vi "scandata.vi"() -> ()   [LabVIEW 2020]
uses:
  <userlib>/Nanonis Prog Interface V5/Nanonis Prog Interface.lvlib
panel:
  in  "function name":string
  in  "module path":path
  in  "Y (m)":sgl min=-0.001 max=0.001 format="%.3p"
  in  "X (m)":sgl min=-0.001 max=0.001 format="%.3p"
  in  "Center coordinates (m)":cluster{"Xc":sgl, "Yc":sgl}={"Xc"=nan, "Yc"=nan} caption="Center coordinates (m) (NaN=no change)" {"Yc" format="%.2p"; "Xc" format="%.2p"}
  in  "Pixels":i32 caption="Pixels/line (0=no change)"
  out "Lines":i32
  out "Pixels/line":i32
  out "Channels indexes (0-23)":i32[](array[numeric])
  in  "Auto save":bool
  in  "Serie name":string="ScanMultiBias_"
  in  "Bias increment":sgl=0.1
  in  "Number of scans":u8=5
  out "Bias voltage":sgl caption="Current bias voltage"
  out "Scan":u8 caption="Current scan"
  out "Saved file path":path
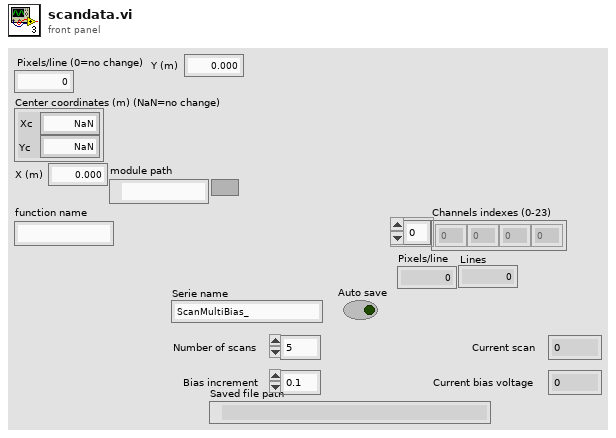
[diagram p1: front panel]
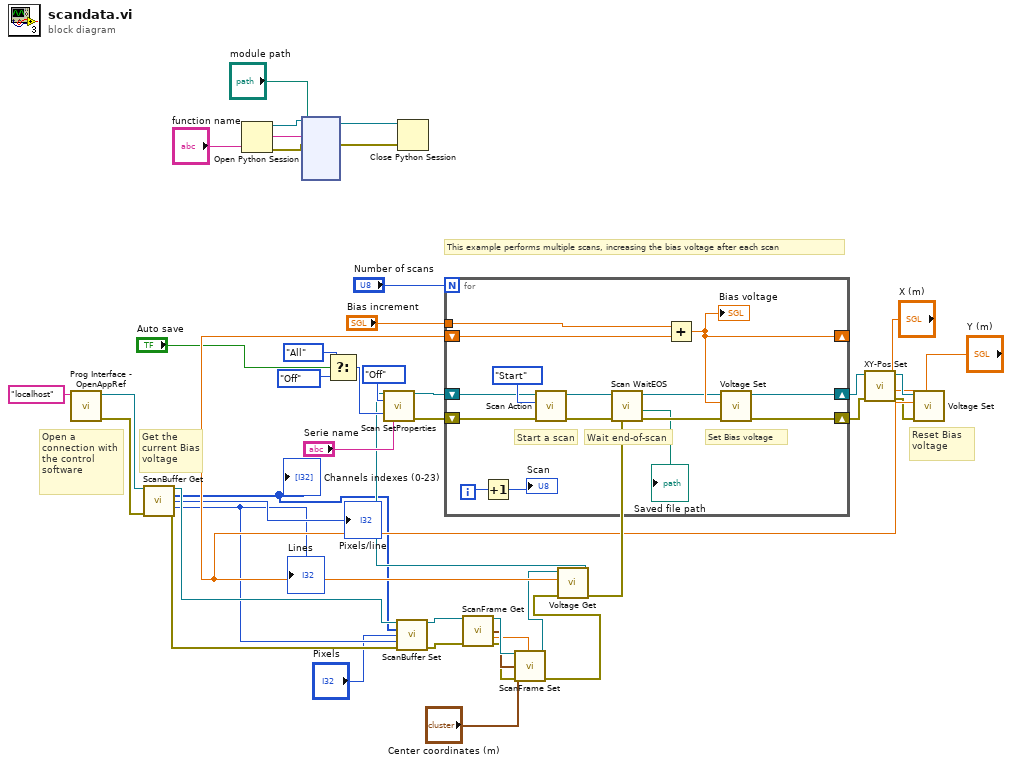
[diagram p0: block diagram]
diagram:
  # "Reset Bias voltage"
  # "Open a connection with the control\nsoftware"
  # "This example performs multiple scans, increasing the bias voltage after each scan"
  # "Get the current Bias voltage"
  n1 = call <userlib>:"Prog Interface - OpenAppRef.vi"("Machine name (local machine IP)"="localhost" ("Machine name (localhost)")) -> ("Error out"=w29:errorcluster, "Application reference"=w28:refnum<vi>)  [unwired: 5 in]
  n2 = call <userlib>:"ScanBuffer Get.vi"("Application ref in"=w28, "error in (no error)"=w29) -> ("Application ref out"=w27:refnum<vi>, "Channels indexes (0-23)"=w25:i32[], "Pixels/line"=→"Pixels/line":i32, "Lines"=w23:i32, "error out"=w26:errorcluster)  [unwired: 9 in]
  "Channels indexes (0-23)" <- w25
  "Lines" <- w23
  n3 = Open Python Session() -> (session out=w6:refnum<k35>, error out=w2:errorcluster)  [unwired: 3 in]
  n4 = node(w6, "module path", "function name", w2) -> (w4:refnum<k35>, w3:errorcluster)  [unwired: 8 in, 2 out]
  n5 = Select(t=enum16{"No change", "All", "Next", "Off"}."All" ("Auto save"), s="Auto save", f=enum16{"No change", "All", "Next", "Off"}."Off" ("Auto save")) -> (s? t:f=w32:enum16{"No change", "All", "Next", "Off"})
  n6 = call <userlib>:"ScanBuffer Set.vi"("Application ref in"=w27, "Channels indexes (0-23)"=w25, "Pixels"="Pixels", "Lines"=w23, "error in (no error)"=w26) -> ("Application ref out"=w21:refnum<vi>, "error out"=w20:errorcluster)  [unwired: 9 in]
  n7 = Close Python Session(session in=w4, error in=w3) -> ()  [unwired: 1 out]
  n8 = call <userlib>:"ScanFrame Get.vi"("Application ref in"=w21, "error in (no error)"=w20) -> ("Application ref out"=w19:refnum<vi>, "Size (m)"=w18:cluster{"Width":sgl, "Height":sgl}, "Angle (deg)"=w17:sgl, "error out"=w16:errorcluster)  [unwired: 9 in, 1 out]
  n9 = call <userlib>:"ScanFrame Set.vi"("Application ref in"=w19, "Center coordinates (m)"="Center coordinates (m)", "Size (m)"=w18, "Angle (deg)"=w17, "error in (no error)"=w16) -> ("Application ref out"=w14:refnum<vi>, "error out"=w15:errorcluster)  [unwired: 9 in]
  n10 = call <userlib>:"Voltage Get.vi"("error in (no error)"=w15, "Application ref in"=w14) -> ("error out"=w40:errorcluster, "Bias (V)"=w37:sgl, "Application ref out"=w31:refnum<vi>)  [unwired: 7 in]
  n11 = call <userlib>:"Scan SetProperties.vi"("Application ref in"=w31, "Continuous scan"=enum16{"No change", "On", "Off"}."Off", "Auto save"=w32, "Error in (no error)"=w40, "Serie name"="Serie name") -> ("Application ref out"=w30:refnum<vi>, "Error out"=w39:errorcluster)  [unwired: 9 in]
  n12 = for {
    N: "Number of scans" -> [_]
    tunnel: "Bias increment" -> [w58]
    shift-right: [w57] -> w11
    shift-left: w39 -> [w54]
    shift-right: [w50] -> _
    shift-left: w37 -> [w51]
    shift-right: [w45] -> w12
    shift-left: w30 -> [w48]
    i -> [w56]
    # "Set Bias voltage"
    # "Wait end-of-scan"
    # "Start a scan"
    n13 = Increment(x=w56) -> (x+1=→"Scan":i32)
    n14 = call <userlib>:"Scan Action.vi"("error in (no error)"=w54, "Scan action (Start)"=enum16{"Start", "Stop", "Pause", "Resume"}."Start" ("Scan action"), "Application ref in"=w48) -> ("error out"=w53:errorcluster, "Application ref out"=w47:refnum<vi>)  [unwired: 6 in]
    n15 = call <userlib>:"Scan WaitEOS.vi"("error in (no error)"=w53, "Application ref in"=w47) -> ("error out"=w52:errorcluster, "Saved file path"=→"Saved file path":path, "Application ref out"=w46:refnum<vi>)  [unwired: 5 in, 1 out]
    n16 = Add(x=w58, y=w51) -> (x+y=w50:sgl)
    "Bias voltage" <- w50
    n17 = call <userlib>:"Voltage Set.vi"("Error in (no error)"=w52, "Bias (V)"=w50, "Application ref in"=w46) -> ("Error out"=w57:errorcluster, "Application ref out"=w45:refnum<vi>)  [unwired: 7 in]
  }
  n18 = call <userlib>:"XY-Pos Set.vi"("error in (no error)"=w11, "Y (m)"="Y (m)", "X (m)"="X (m)", "Application ref in"=w12) -> ("error out"=w9:errorcluster, "Application ref out"=w10:refnum<vi>)  [unwired: 4 in]
  n19 = call <userlib>:"Voltage Set.vi"("Error in (no error)"=w9, "Bias (V)"=w37, "Application ref in"=w10) -> ()  [unwired: 7 in, 2 out]
